vi "Read Inputs from system.vi"(8 "error in":errorcluster, 11 "Custom Controller Module runtime in":refnum<class "Custom Controller Module runtime.lvclass">) -> (0 "error out":errorcluster, 2 "Inputs from system":T1, 3 "Custom Controller Module runtime out":refnum<class "Custom Controller Module runtime.lvclass">)   [LabVIEW 2013, in "Custom Controller Module runtime.lvclass"]
uses:
  Custom Controller Module runtime.lvclass
  configuration/input data indices.ctl
  Custom Controller Module runtime.lvclass/Custom Controller Module runtime.ctl
  configuration/Custom Controller Module configuration.lvclass
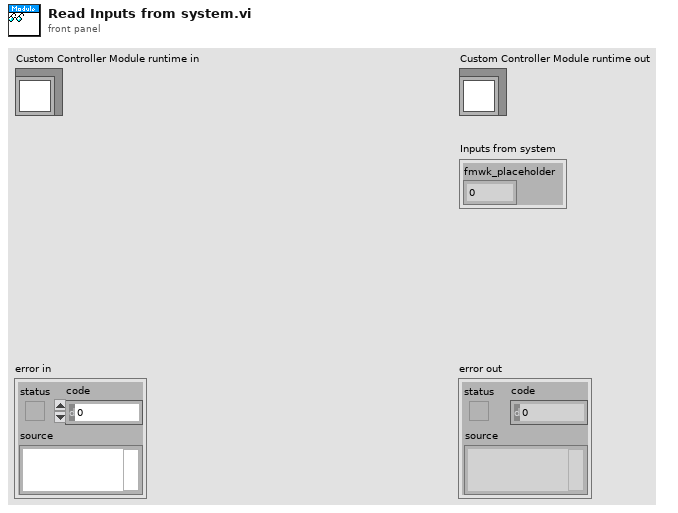
[diagram p1: front panel]
types:
  T1 = typedef "Custom Controller Module configuration.lvclass/input data indices.ctl" = cluster{"fmwk_placeholder":i32}
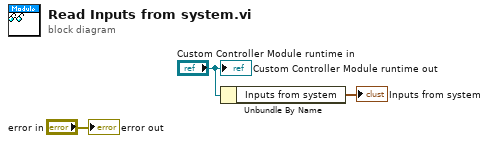
[diagram p0: block diagram]
diagram:
  n1 = Unbundle By Name("Custom Controller Module runtime in") -> ("Inputs from system"=→"Inputs from system":T1)
  "error out" <- "error in"
  "Custom Controller Module runtime out" <- "Custom Controller Module runtime in"
